vi "ImageHistogram.vi"(11 "image data":T2) -> (3 "Histogram Graph":T1)   [LabVIEW 2019]
uses:
  <vilib>/picture/picture.llb/imagedata.ctl
  Histograph.ctl
  <vilib>/Analysis/NI_AALPro.lvlib
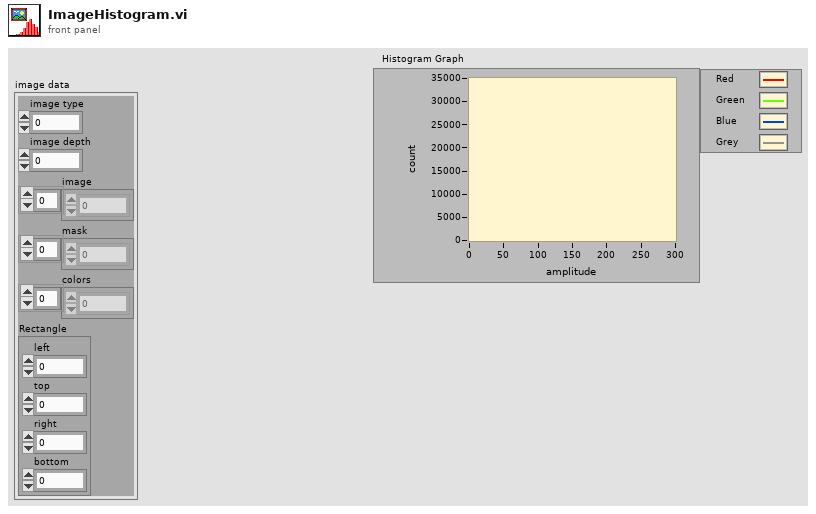
[diagram p1: front panel]
types:
  T1 = typedef "Histograph.ctl" = cluster{"X Values":dbl[], "Histogram: h(x)":i32[]}[]
  T2 = typedef "imagedata.ctl" = cluster{"image type":i32, "image depth":i32, "image":u8[], "mask":u8[], "colors":u32[], "Rectangle":cluster{"left":i16, "top":i16, "right":i16, "bottom":i16}}
  T3 = cluster{"X Values":dbl[], "Histogram: h(x)":i32[]}
  T4 = cluster{"X Values":dbl[], "Histogram: h(x)":i32[]}[]
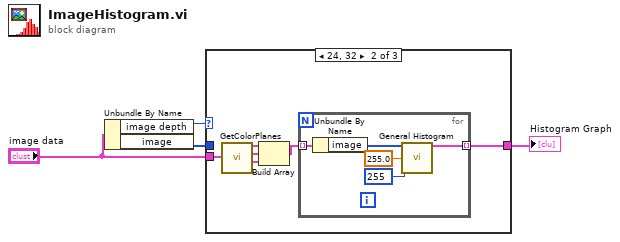
[diagram p0: block diagram]
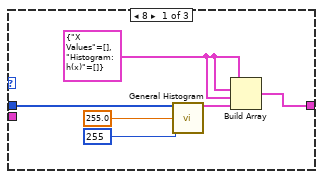
[diagram p2: hidden frame]
diagram:
  n1 = Unbundle By Name("image data") -> ("image depth"=w4:i32, "image"=w3:u8[])
  n2 = case shown="24, 32" w4 {
    tunnel: w3 -> [w10 _ _]
    tunnel: [w6 w16 _] -> w2
    tunnel: "image data" -> [_ w14 _]
    frame 8 {
      w5 = T3 {"X Values"=[], "Histogram: h(x)"=[]} ("Histogram Graph")
      n3 = call <vilib>:"General Histogram.vi"("X"=w10, "max"=255.0, "# bins"=255) -> ("Histogram Graph"=w7:T3)  [unwired: 8 in, 4 out]
      n4 = Build Array(w5, w5, w5, w7) -> (w6:T4)
    }
    frame 24, 32 {
      n5 = call "GetColorPlanes.vi"("image data"=w14) -> ("Blue"=w11:T2, "Green"=w12:T2, "Red"=w13:T2)  [unwired: 7 in, 1 out]
      n6 = Build Array(w13, w12, w11) -> (w15:T2[])
      n7 = for {
        tunnel: [w19] -> w16 mode=indexing
        tunnel: w15 -> [w18] mode=indexing
        n8 = Unbundle By Name(w18) -> ("image"=w17:u8[])
        n9 = call <vilib>:"General Histogram.vi"("X"=w17, "max"=255.0, "# bins"=255) -> ("Histogram Graph"=w19:T3)  [unwired: 8 in, 4 out]
      }
    }
    frame Default {
    }
  }
  "Histogram Graph" <- w2
